vi "test_db_variable.vi"(10 "Action":T1, 11 "Test DB in":bool) -> (2 "Test DB out":bool)   [LabVIEW 2013]
uses:
  Action Items.ctl
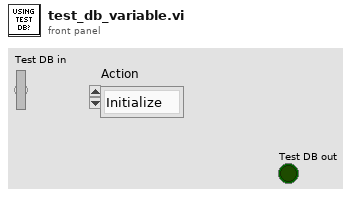
[diagram p1: front panel]
types:
  T1 = typedef "Action Items.ctl" = enum16{"Initialize", "Get", "Set"}
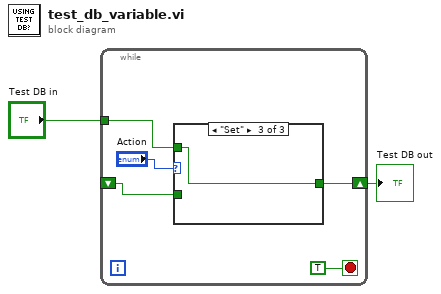
[diagram p0: block diagram]
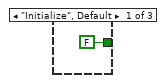
[diagram p2: hidden frame]
diagram:
  n1 = while {
    shift-right: [w4] -> w1
    shift-left: _ -> [w3]
    tunnel: "Test DB in" -> [w5]
    stop <- TRUE stop-if-true
    n2 = case shown="\"Set\"" "Action" {
      tunnel: w5 -> [_ _ w10]
      tunnel: [FALSE ("Test DB?") w9 w10] -> w4
      tunnel: w3 -> [_ w9 _]
      frame "Initialize", Default {
      }
      frame "Get" {
      }
      frame "Set" {
      }
    }
  }
  "Test DB out" <- w1
